vi "Read ROI.vi"(8 "error in (no error)":errorcluster, 11 "CameraSession in":refnum<class "CameraSession.lvclass">) -> (0 "error out":errorcluster, 2 "ROI":T1, 3 "CameraSession out":refnum<class "CameraSession.lvclass">)   [LabVIEW 2013, in "CameraSession.lvclass"]
uses:
  CameraSession.lvclass
  TypeDefs/rgn_array.ctl
  CameraSession.lvclass/CameraSession.ctl
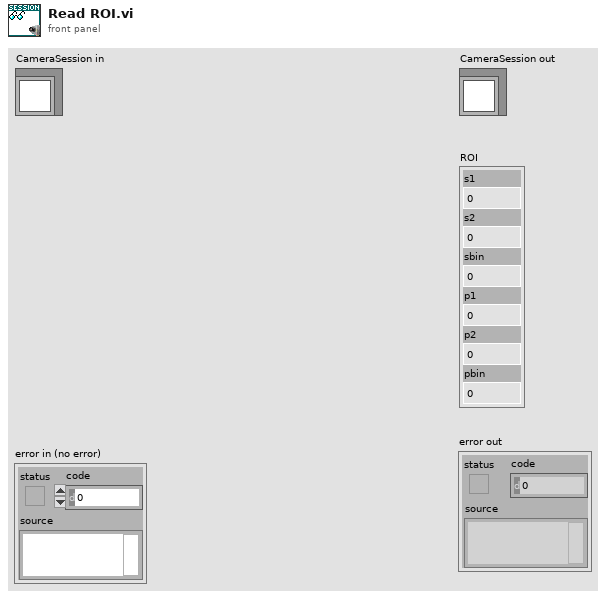
[diagram p1: front panel]
types:
  T1 = typedef "rgn_array.ctl" = cluster{"s1":u16, "s2":u16, "sbin":u16, "p1":u16, "p2":u16, "pbin":u16}
  T2 = cluster{"s1":u16, "s2":u16, "sbin":u16, "p1":u16, "p2":u16, "pbin":u16}
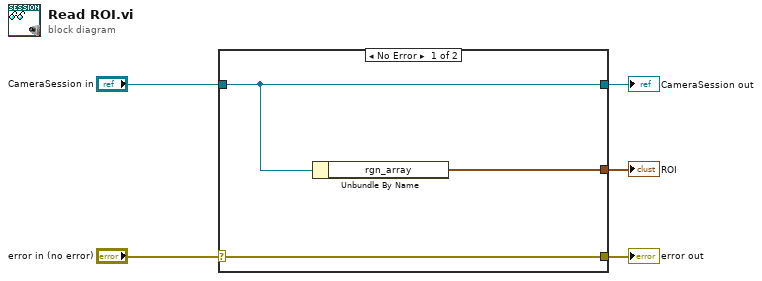
[diagram p0: block diagram]
diagram:
  n1 = case shown="No Error" "error in (no error)" {
    selector: "error in (no error)" -> [w8 w9]
    tunnel: [w8 w9] -> w4
    tunnel: [w7 w10] -> w2
    tunnel: "CameraSession in" -> [w7 w10]
    tunnel: [w6 _] -> w1
    frame No Error {
      n2 = Unbundle By Name(w7) -> ("rgn_array"=w6:T2)
    }
    frame Error {
    }
  }
  "error out" <- w4
  "CameraSession out" <- w2
  "ROI" <- w1
